vi "EEPROM INI Read.vi"(3 "error in (no error)":errorcluster, 4 "Path":path) -> (0 "error out":errorcluster, 1 "EEPROM Data":T1)   [LabVIEW 2010, in "lib1299.lvlib"]
doc: "This VI reads the EEPROM programming information (device and EDGE numbers) from the \"EEPROM_EVM.ini\" file located within the same directory as this VI.\n\nInputs:\nerror in - error input cluster\n\nOutputs:\nEEPROM Data - cluster of strings read from the ini file\n => EVM Name - name of the EVM\n => PWB EDGE No. - EDGE number for the PWB\n => PCA EDGE No. - EDGE number for the PCA\n => BOM EDGE No. - EDGE number for the BOM"
uses:
  lib1299.lvlib
  Controls/EEPROM_data.ctl
  Controls/EDGE ITEM.ctl
  <vilib>/Utility/config.llb/Read Key (String).vi
  <vilib>/Utility/config.llb/NI_LVConfig.lvlib
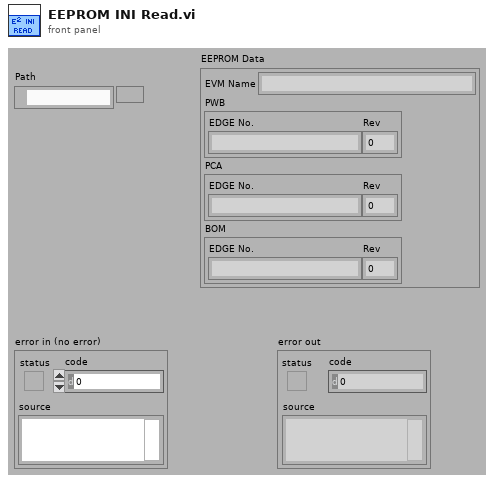
[diagram p1: front panel]
types:
  T1 = typedef "lib1299.lvlib/EEPROM_data.ctl" = cluster{"EVM Name":string, "PWB":T2, "PCA":T2, "BOM":T2}
  T2 = typedef "lib1299.lvlib/EDGE ITEM.ctl" = cluster{"EDGE No.":string, "Rev":u16}
  T3 = typedef "NI_LVConfig.lvlib/Config Data RefNum.ctl" = refnum<k1>
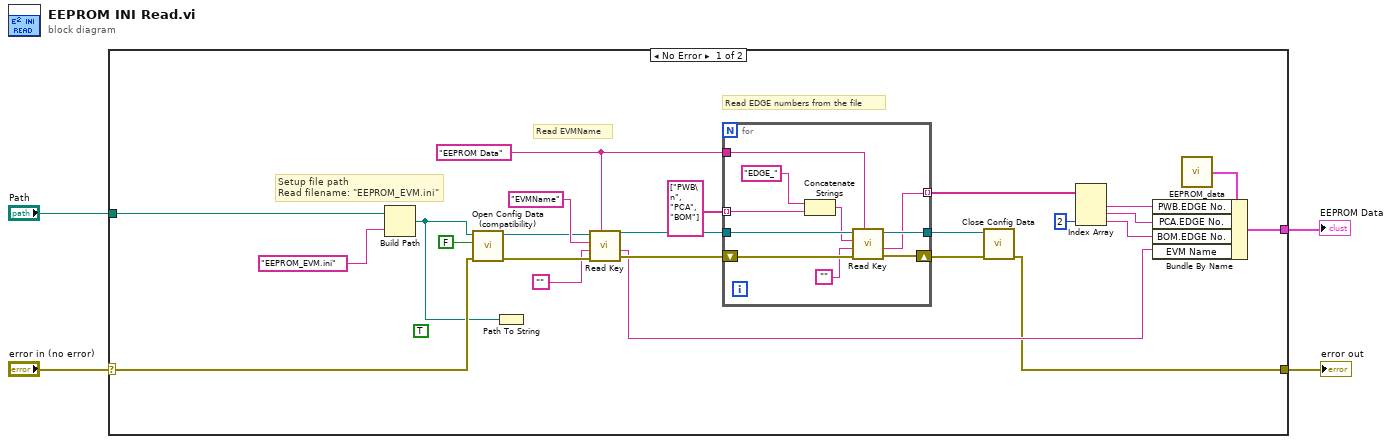
[diagram p0: block diagram]
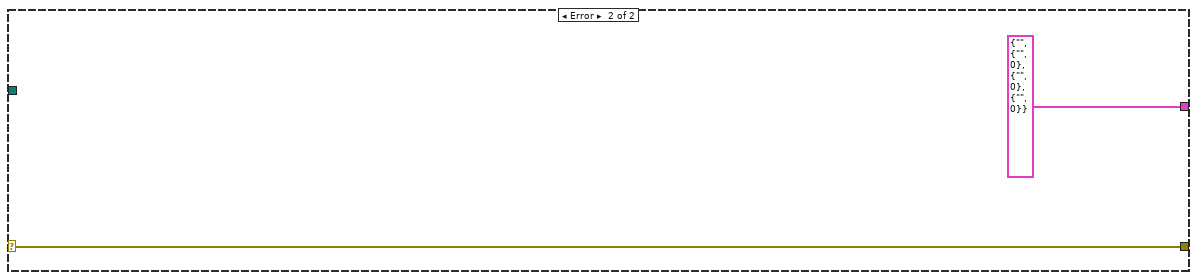
[diagram p2: hidden frame]
diagram:
  n1 = case shown="No Error" "error in (no error)" {
    selector: "error in (no error)" -> [w28 w40]
    tunnel: [w7 w40] -> w3
    tunnel: [w17 T1 {"EVM Name"="", "PWB"={"EDGE No."="", "Rev"=0}, "PCA"={"EDGE No."="", "Rev"=0}, "BOM"={"EDGE No."="", "Rev"=0}} ("EEPROM Data")] -> w2
    tunnel: "Path" -> [w6 _]
    frame No Error {
      (unwired) TRUE ("create file if necessary? (T)")
      w10 = "EEPROM Data"
      # "Read EDGE numbers from the file"
      # "Read EVMName"
      # "Setup file path\nRead filename: \"EEPROM_EVM.ini\""
      n2 = Build Path(base path=w6, name or relative path="EEPROM_EVM.ini") -> (appended path=w5:path)
      n3 = call <vilib>:"Open Config Data (compatibility).vi"("error in (no error)"=w28, "create file if necessary (T)"=FALSE ("create file if necessary? (T)"), "configuration file path"=w5) -> ("error out"=w25:errorcluster, "refnum"=w11:T3)  [unwired: 6 in, 1 out]
      n4 = Path To String(path=w5) -> ()  [unwired: 1 out]
      n5 = call-poly <vilib>:"Read Key.vi"("section"=w10, "error in (no error)"=w25, "default value"="", "key"="EVMName" ("name or relative path"), "refnum"=w11) -> ("error out"=w23:errorcluster, "value"=w18:string, "refnum out"=w24:T3)  [unwired: 3 in, 1 out]
      n6 = for {
        tunnel: w24 -> [w38]
        tunnel: [w36] -> w9
        tunnel: w10 -> [w34]
        shift-right: [w35] -> w8
        shift-left: w23 -> [w33]
        tunnel: string[] ["PWB\n", "PCA", "BOM"] -> [w31] mode=indexing
        tunnel: [w30] -> w16 mode=indexing
        n7 = Concatenate Strings("EDGE_" ("name or relative path"), w31) -> (w37:string)
        n8 = call-poly <vilib>:"Read Key.vi"("section"=w34, "error in (no error)"=w33, "default value"="", "key"=w37, "refnum"=w38) -> ("error out"=w35:errorcluster, "value"=w30:string, "refnum out"=w36:T3)  [unwired: 3 in, 1 out]
      }
      n9 = call <vilib>:"Close Config Data.vi"("error in (no error)"=w8, "refnum"=w9) -> ("error out"=w7:errorcluster)  [unwired: 8 in, 1 out]
      n10 = Index Array(array=w16, index #3=2 ("index")) -> (element #1=w12:string, element #2=w13:string, element #3=w14:string)  [unwired: 2 in]
      n11 = call "EEPROM_data.vi"() -> ("EEPROM Data"=w19:T1)  [unwired: 1 in]
      n12 = Bundle By Name(cluster=w19, "PWB.EDGE No."=w12, "PCA.EDGE No."=w13, "BOM.EDGE No."=w14, "EVM Name"=w18) -> (w17:T1)
    }
    frame Error {
    }
  }
  "error out" <- w3
  "EEPROM Data" <- w2
